vi "send_command_no_response.vi"(4 "error in":errorcluster, 5 "Timeout ms (25000)":i32=20000, 6 "JSON Command":string, 7 "TCP Network Connection in":refnum<k5>) -> (0 "error out":errorcluster, 3 "TCP Network Connection Out":refnum<k5>)   [LabVIEW 2019, in "Lib_Simx.lvlib"]
doc: "Send a command via TCP with format \"type\", \"success\", \"reference\", \"message\". This VI is used to send server commands without waiting for the response of the server."
uses:
  Lib_Simx.lvlib
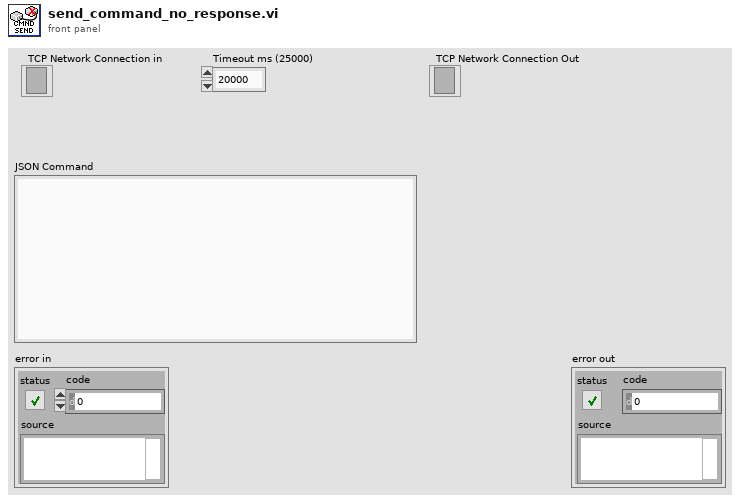
[diagram p1: front panel]
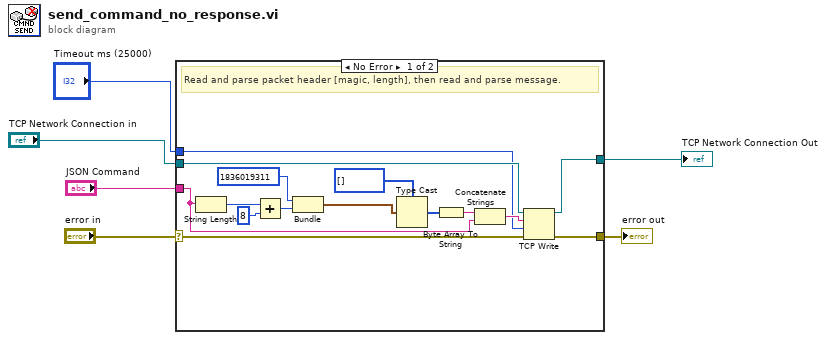
[diagram p0: block diagram]
diagram:
  n1 = case shown="No Error" "error in" {
    selector: "error in" -> [w10 w23]
    tunnel: "TCP Network Connection in" -> [w13 w22]
    tunnel: "JSON Command" -> [w12 _]
    tunnel: [w8 w23] -> w3
    tunnel: [w7 w22] -> w2
    tunnel: "Timeout ms (25000)" -> [w9 _]
    frame No Error {
      # "Read and parse packet header [magic, length], then read and parse message."
      n2 = String Length(string=w12) -> (length=w14:i32)
      n3 = Add(x=w14, y=u32 8) -> (x+y=w16:u32)
      n4 = Bundle(u32 1836019311, w16) -> (w21:cluster{u32, u32})  [unwired: 1 in]
      n5 = Type Cast(type=u8[] [], x=w21) -> (*(type *) &x=w19:u8[])
      n6 = Byte Array To String(unsigned byte array=w19) -> (string=w15:string)
      n7 = Concatenate Strings(w15, w12) -> (w11:string)
      n8 = TCP Write(connection ID=w13, data in=w11, error in (no error)=w10, 9:w9) -> (connection ID out=w7:refnum<k5>, error out=w8:errorcluster)  [unwired: 1 out]
    }
    frame Error {
    }
  }
  "error out" <- w3
  "TCP Network Connection Out" <- w2
